vi "Store VI and FP References.vi"(8 "error in (no error)":errorcluster, 11 "GUI View in":refnum<class "GUI View.lvclass">) -> (0 "error out":errorcluster, 3 "GUI View out":refnum<class "GUI View.lvclass">)   [LabVIEW 2023, in "GUI Views.lvlib" / "GUI View.lvclass"]
uses:
  GUI View.lvclass
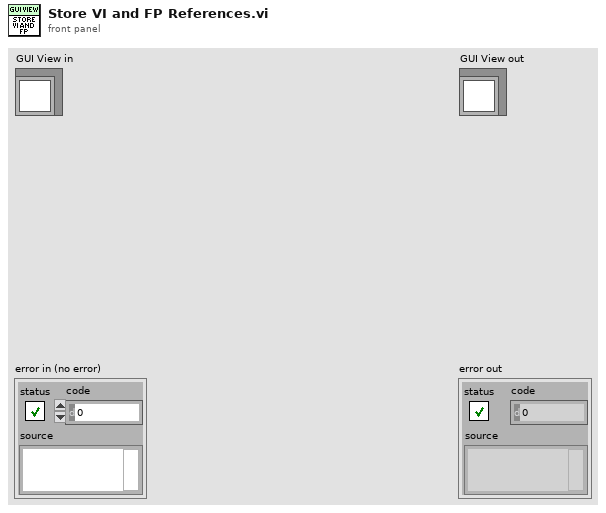
[diagram p1: front panel]
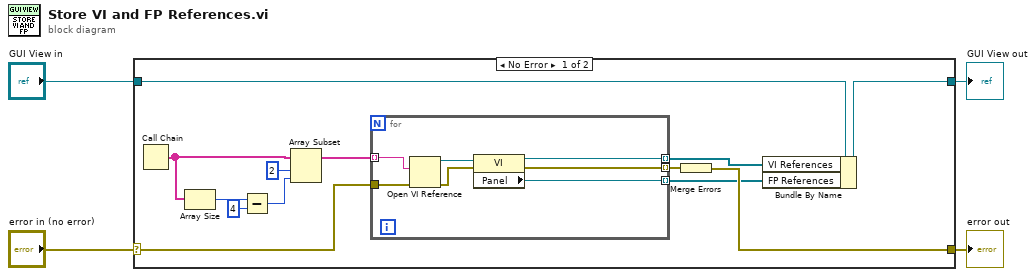
[diagram p0: block diagram]
diagram:
  n1 = case shown="No Error" "error in (no error)" {
    selector: "error in (no error)" -> [w14 w26]
    tunnel: [w13 w26] -> w3
    tunnel: [w12 w25] -> w1
    tunnel: "GUI View in" -> [w17 w25]
    frame No Error {
      n2 = Call Chain() -> (call chain=w8:string[])
      n3 = Array Size(array=w8) -> (size(s)=w7:i32)
      n4 = Subtract(x=w7, y=4) -> (x-y=w5:i32)
      n5 = Array Subset(array=w8, index=2, length=w5) -> (w16:string[])
      n6 = for {
        tunnel: w16 -> [w23] mode=indexing
        tunnel: w14 -> [w24]
        tunnel: [w19] -> w11 mode=indexing
        tunnel: [w20] -> w10 mode=indexing
        tunnel: [w18] -> w9 mode=indexing
        n7 = Open VI Reference(vi path=w23, error in (no error)=w24) -> (vi reference=w22:refnum<vi>, error out=w21:errorcluster)  [unwired: 4 in]
        n8 = property class="VI"(reference=w22, error in=w21) -> (reference out=w18:refnum<vi>, error out=w19:errorcluster, "Panel"=w20:refnum<vi>)
      }
      n9 = Merge Errors(w11) -> (w13:errorcluster)
      n10 = Bundle By Name(cluster=w17, "VI References"=w9, "FP References"=w10) -> (w12:refnum<class "GUI View.lvclass">)
    }
    frame Error {
    }
  }
  "error out" <- w3
  "GUI View out" <- w1
